vi "FRCts20_Backend_Division_PPD_reform.vi"(7 "Division":T1, 8 "error in (no error)":errorcluster, 11 "rows affected":i32) -> (0 "error out":errorcluster, 3 "data string":string)   [LabVIEW 2013]
uses:
  FRCts20_Backend_API/FRCts20_Backend_API_Division.ctl
  FRCts20_Backend_API/FRCts20_Backend_API_SW.ctl
  FRCts20_Backend_API/FRCts20_Backend_API_Status.ctl
  FRCts20_Backend_Engine.lvlib
  FRCts20_Backend_API/FRCts20_Backend_API.lvlib
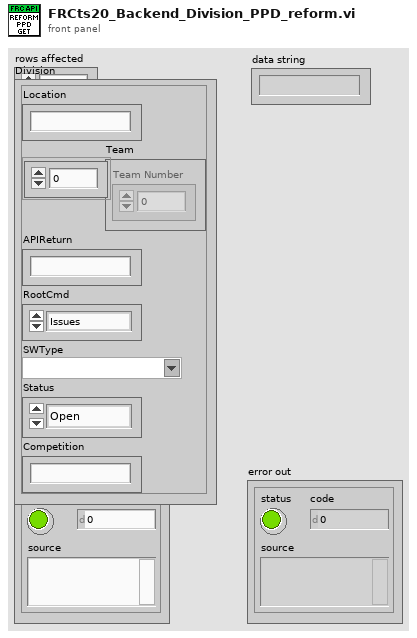
[diagram p1: front panel]
types:
  T1 = typedef "FRCts20_Backend_API.lvlib/FRCts20_Backend_API_Division.ctl" = cluster{"Location":string, "Team":u32[], "APIReturn":string, "RootCmd":enum16{"Issues", "Software", "All"}, "SWType":T2, "Status":T3, "Competition":string}
  T2 = typedef "FRCts20_Backend_API.lvlib/FRCts20_Backend_API_SW.ctl" = string
  T3 = typedef "FRCts20_Backend_API.lvlib/FRCts20_Backend_API_Status.ctl" = enum16{"Open", "In Work", "Closed"}
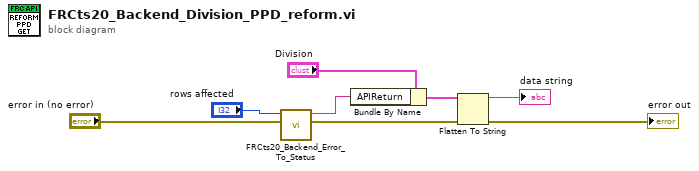
[diagram p0: block diagram]
diagram:
  n1 = call "FRCts20_Backend_Error_To_Status.vi"("error in (no error)"="error in (no error)", "rows affected"="rows affected") -> ("error out"=w4:errorcluster, "String"=w5:string)  [unwired: 8 in]
  n2 = Bundle By Name(cluster="Division", "APIReturn"=w5) -> (w1:T1)
  n3 = Flatten To String(anything=w1, error in (no error)=w4) -> (data string=→"data string":string, error out=→"error out":errorcluster)  [unwired: 2 in, 1 out]
